vi "条件禁用.vi"(9 "远程":bool, 10 "state":string="整流器柜BOOL", 11 "队列输入":refnum<queue>) -> ()   [LabVIEW 2015]
uses:
  <userlib>/QMH/Message Queue/Support/Message Cluster.ctl
  <userlib>/QMH/Message Queue/Support/Enqueue Message (Single).vi
  <userlib>/QMH/Message Queue/Message Queue.lvlib
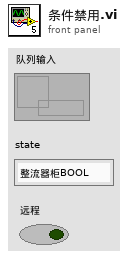
[diagram p1: front panel]
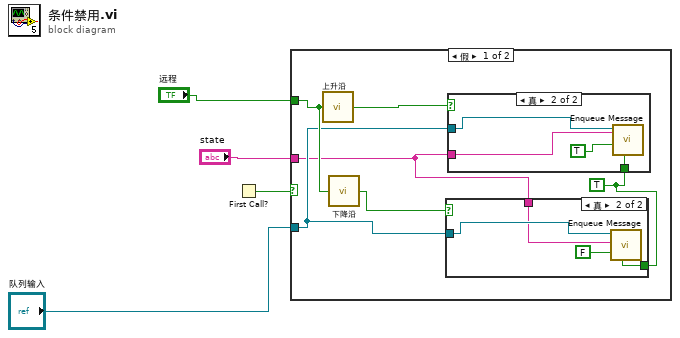
[diagram p0: block diagram]
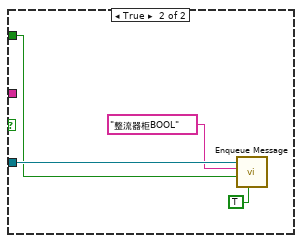
[diagram p4: hidden frame]
diagram:
  n1 = First Call?() -> (First Call?: T/F=w3:bool)
  n2 = case shown="假" w3 {
    tunnel: "队列输入" -> [w7 w22]
    tunnel: "远程" -> [w9 w20]
    tunnel: "state" -> [w6 _]
    frame False {
      w5 = TRUE
      n3 = call "上升沿.vi"("Boolean Input"=w9) -> ("Rising Edge"=w10:bool)
      n4 = call "下降沿.vi"("Boolean Input"=w9) -> ("Falling Edge"=w8:bool)
      n5 = case shown="真" w8 {
        tunnel: w7 -> [_ w14]
        tunnel: w6 -> [_ w12]
        tunnel: w5 -> [_ w11]
        frame False {
        }
        frame True {
          n6 = call-poly <userlib>:"Enqueue Message.vi"("Priority Message? (F)"=w11, "Message Data"=FALSE, "Message"=w12, "Message Queue"=w14) -> ()  [unwired: 6 in, 2 out]
        }
      }
      n7 = case shown="真" w10 {
        tunnel: w7 -> [_ w18]
        tunnel: w6 -> [_ w16]
        tunnel: w5 -> [_ w15]
        frame False {
        }
        frame True {
          n8 = call-poly <userlib>:"Enqueue Message.vi"("Priority Message? (F)"=w15, "Message Data"=TRUE, "Message"=w16, "Message Queue"=w18) -> ()  [unwired: 6 in, 2 out]
        }
      }
    }
    frame True {
      n9 = call-poly <userlib>:"Enqueue Message.vi"("Priority Message? (F)"=TRUE, "Message Data"=w20, "Message"="整流器柜BOOL" ("state"), "Message Queue"=w22) -> ()  [unwired: 6 in, 2 out]
    }
  }
